vi "Do.vi"(8 "error in (no error)":errorcluster, 10 "Actor in":refnum<class "Actor.lvclass">, 11 "Send Message Msg in":refnum<class "Send Message Msg.lvclass">) -> (0 "error out":errorcluster, 2 "Actor out":refnum<class "Actor.lvclass">)   [LabVIEW 2017, in "WebSocket Client.lvlib" / "Send Message Msg.lvclass"]
doc: "This VI delivers the message to the actor by calling the appropriate method(s) on the actor."
uses:
  Send Message Msg.lvclass
  <vilib>/ActorFramework/Actor/Actor.lvclass
  WebSocket Client/WebSocket Client.lvclass
  Applications/National Instruments/LabVIEW 2017 64-bit/vi.lib/ActorFramework/Actor/Actor.lvclass
  Send Message Msg.lvclass/Send Message Msg.ctl
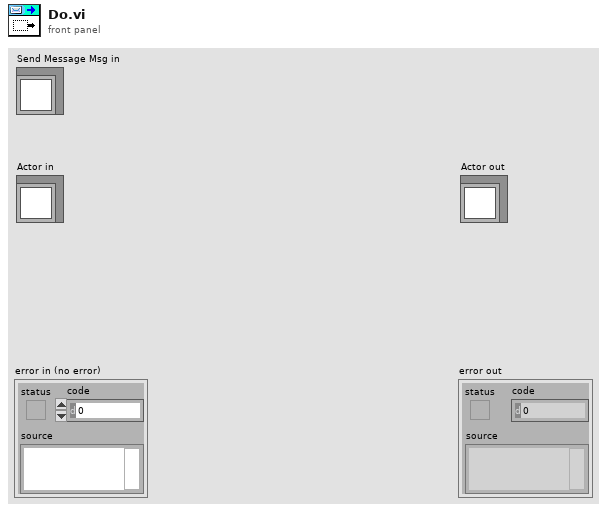
[diagram p1: front panel]
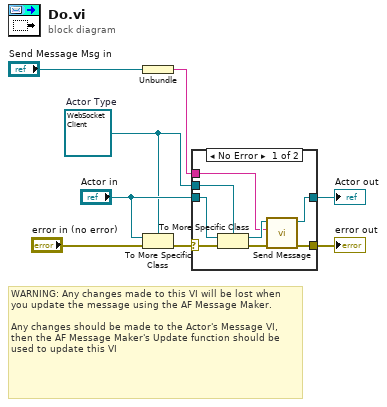
[diagram p0: block diagram]
diagram:
  w3 = refnum<class "WebSocket Client.lvclass"> refnum  # Actor Type
  # "WARNING: Any changes made to this VI will be lost when you update the message using the AF Message Maker.\n\nAny changes should be made to the Actor's Message VI, then the AF Message Maker's Update function should be used to update this VI"
  n1 = Unbundle("Send Message Msg in") -> (w2:string)
  n2 = To More Specific Class(target class=w3, reference="Actor in", error in="error in (no error)") -> (error out=w7:errorcluster)  [unwired: 1 out]
  n3 = case shown="No Error" w7 {
    selector: w7 -> [w16 w18]
    tunnel: [w11 w18] -> w6
    tunnel: [w10 w17] -> w5
    tunnel: "Actor in" -> [w15 w17]
    tunnel: w3 -> [w14 _]
    tunnel: w2 -> [w9 _]
    frame No Error {
      n4 = To More Specific Class ("Actor Cast")(target class=w14, reference=w15, error in=w16) -> (specific class reference=w13:refnum<class "WebSocket Client.lvclass">, error out=w12:errorcluster)
      n5 = call "Send Message.vi"("error in (no error)"=w12, "Message"=w9, "WebSocket Client in"=w13) -> ("error out"=w11:errorcluster, "WebSocket Client out"=w10:refnum<class "WebSocket Client.lvclass">)  [unwired: 7 in]
    }
    frame Error {
    }
  }
  "error out" <- w6
  "Actor out" <- w5
